vi "LDA_Analysis_1.vi"() -> (5 "Plug in titles":string[](array[string]), 7 "Plug in values":string[](array[string]))   [LabVIEW 2010]
uses:
  Globals/Plug_in_data_global.vi
  Globals/LDA_meas_global_1.vi
  Globals/Meas_global.vi
  Globals/Constants_global.vi
  Controls/Save_Data.ctl
  <vilib>/Analysis/NI_AALBase.lvlib
panel:
  in  "No of estimates output":i32=300
  out "Autocorrelation":cluster{dbl, dbl, dbl[]}[](graph)
  in  "Mode":T1(ring)
  in  "Separation Character":string="\t"
  in  "Precision":i16=2
  out "Ch names":string[](array[string])
  out "Number or Good blocks":i32
  out "Resampled block length":i32
  out "Resampling Frequency":dbl
  in  "Output Directory":path
  in  "File":T2=enum."Save Data"
  out "Frequency Spectrum":cluster{dbl, dbl, dbl[]}[](graph)
  # "You must have just these two indicators on the connector pane of the vi"
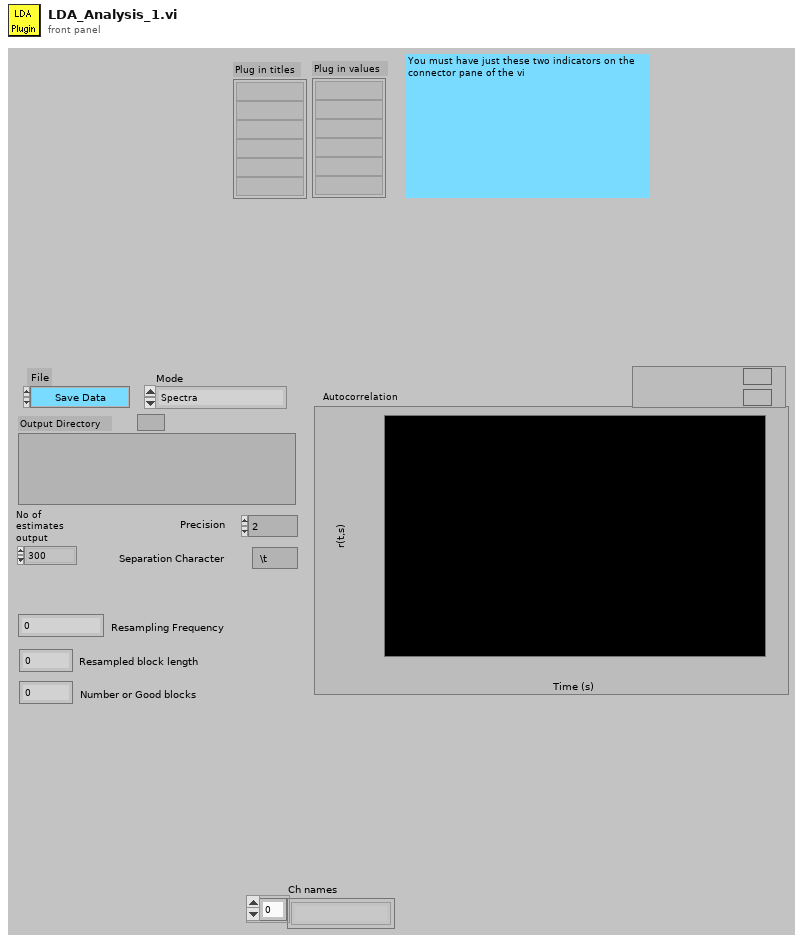
[diagram p1: front panel]
types:
  T1 = enum16{"Spectra", "Autocorrelation", "Calculate Error bars"}
  T2 = typedef "Save_Data.ctl" = enum16{"Save No Data", "Save Data"}
  T3 = enum32{"existing file", "new file", "new or existing file", "existing dir", "new dir", "new or existing dir", "existing file (use LLBs)", "new file (use LLBs)", "new or existing file (use LLBs)", "new or existing file or directory (use LLBs)"}
  T4 = typedef "Analysis_info_cluster.ctl" = cluster{"Colour":u32, "Inst type":T5, "Inst name":string, "Symbol":string, "Code name":string, "Extra Info":string, "Inst Array":T6, "Index":i32, "Voltage Index":i32, "Extra Titles":string[], "Extra Values":string[]}
  T5 = typedef "Inst_type.ctl" = enum16{"Propeller anemometer", "Raw voltage", "Pressure Transducer", "Pitot-static tube", "Preston tube", "Hot wire", "Cross wire 1", "Cross wire 2", "Generic Linear", "Generic Polynomial", "Generic BackPoly", "Fast FID", "Thermocouple", "Cold wire", "Pulsed Wire", "LDA Vel", "LDA Tran time", "LDA Arr time"}
  T6 = typedef "Instrument_Array.ctl" = enum16{"PWA", "LDA", "Analogue"}
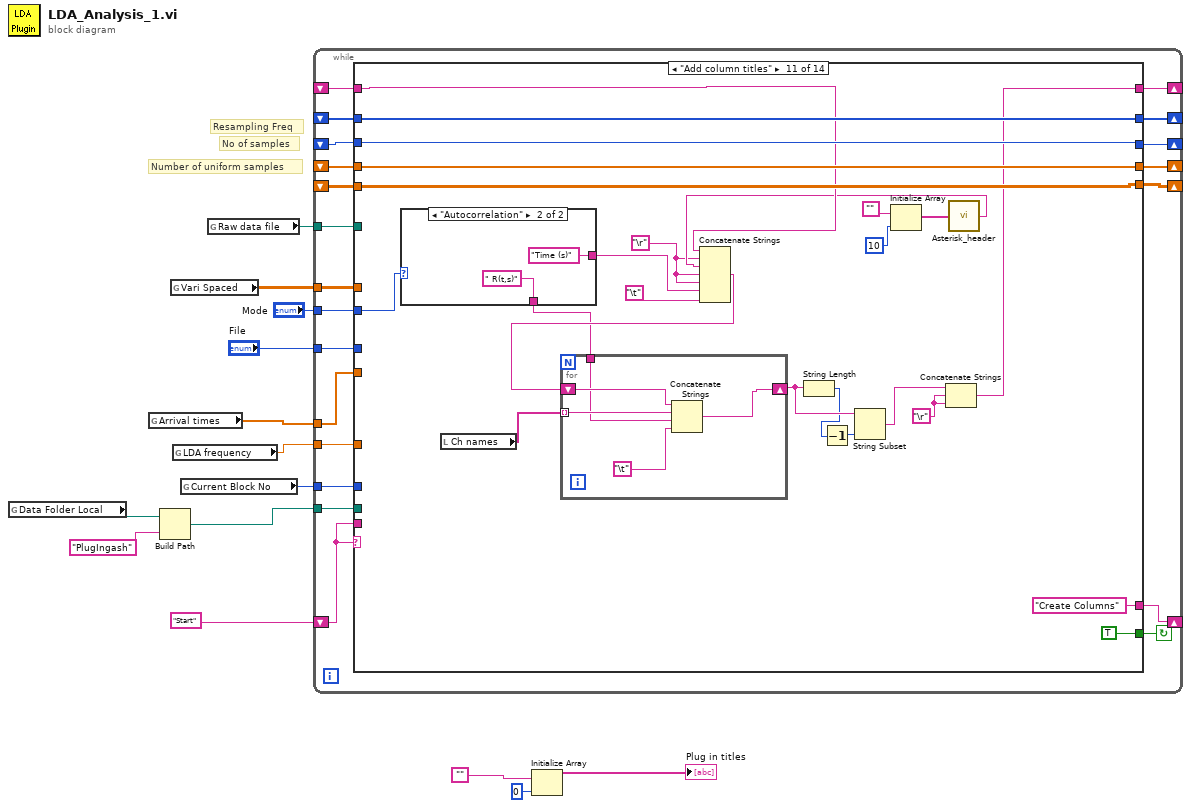
[diagram p0: block diagram]
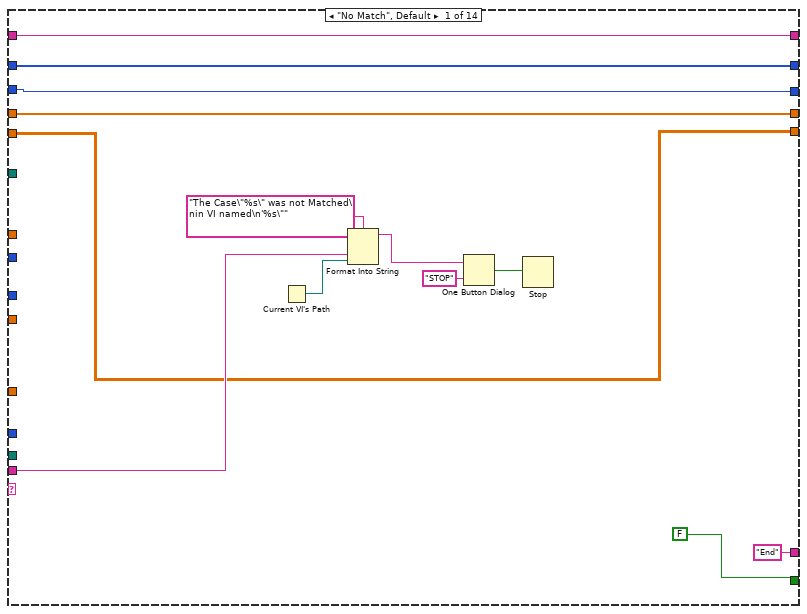
[diagram p2: hidden frame]
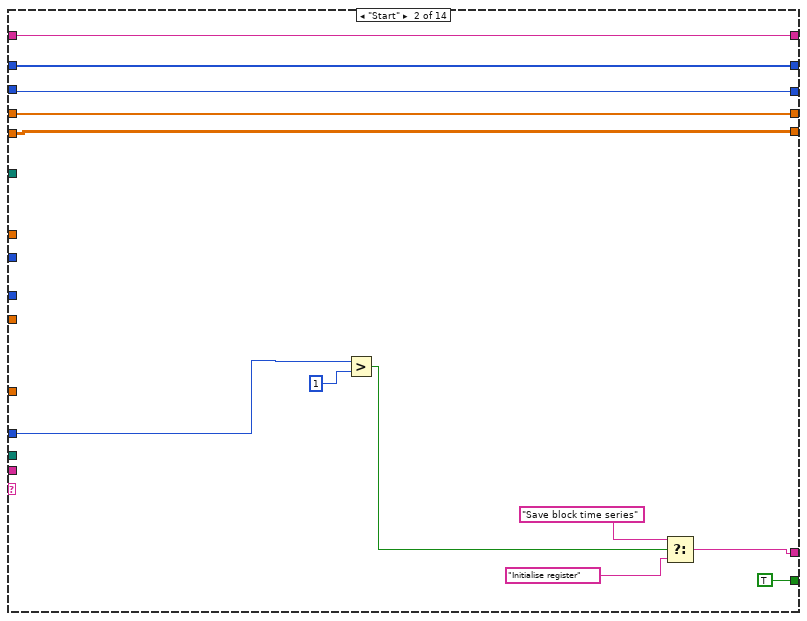
[diagram p3: hidden frame]
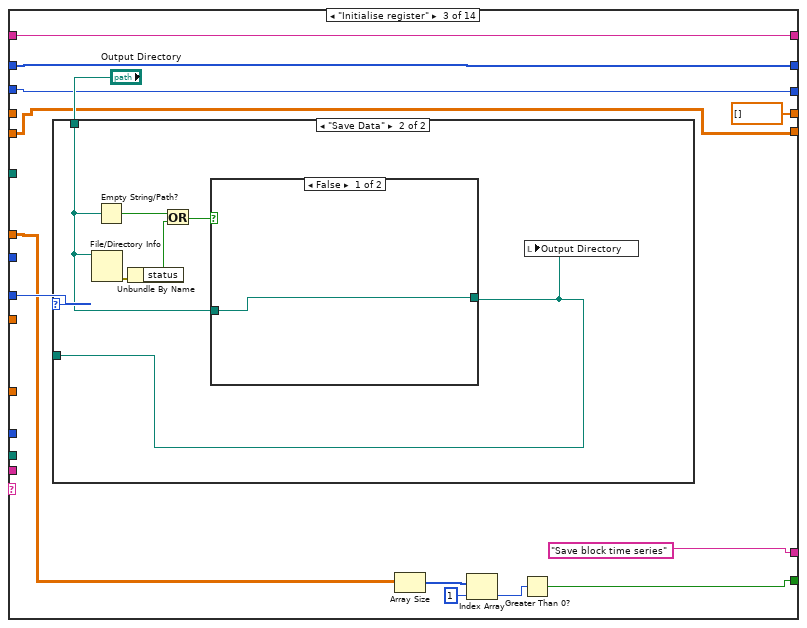
[diagram p4: hidden frame]
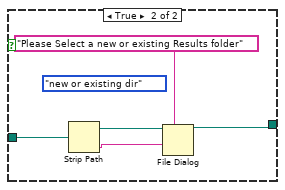
[diagram p6: hidden frame]
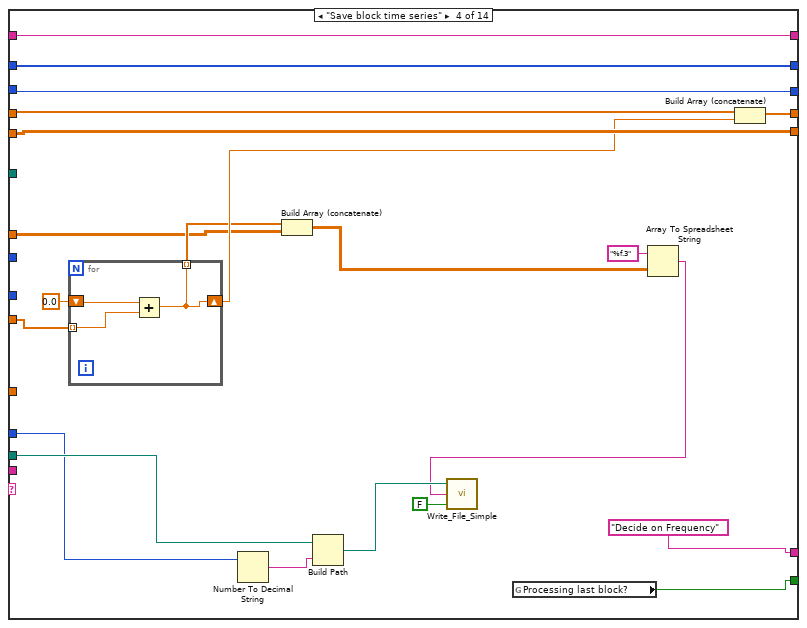
[diagram p7: hidden frame]
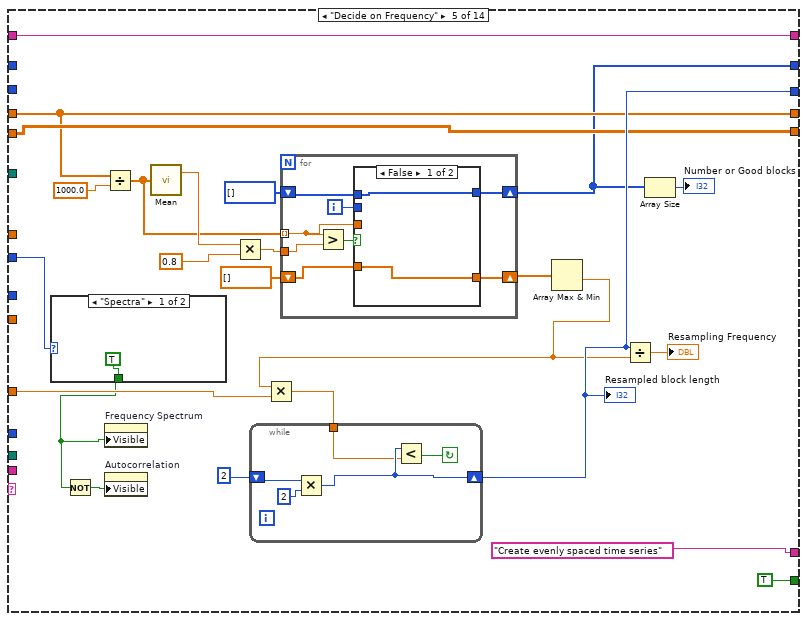
[diagram p8: hidden frame]
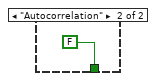
[diagram p9: hidden frame]
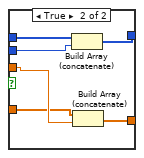
[diagram p10: hidden frame]
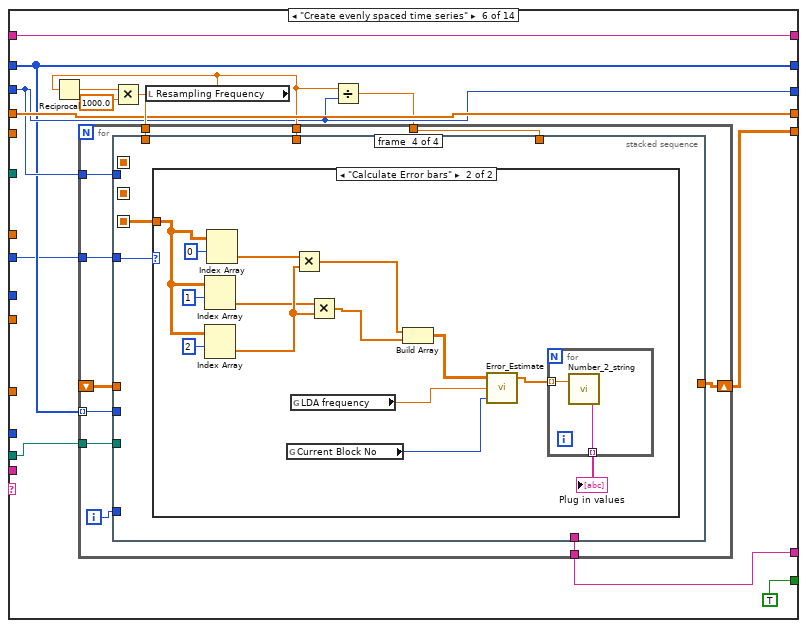
[diagram p11: hidden frame]
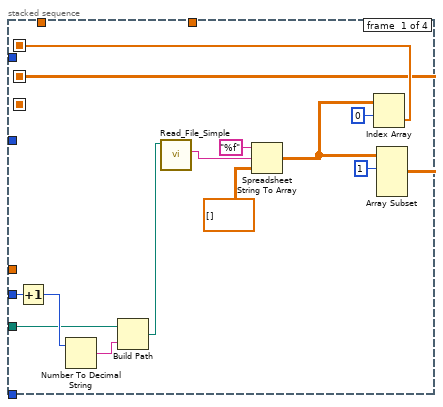
[diagram p12: hidden frame]
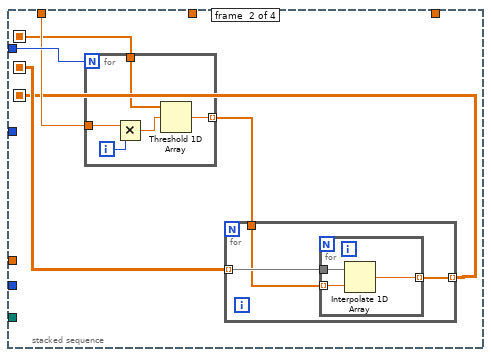
[diagram p13: hidden frame]
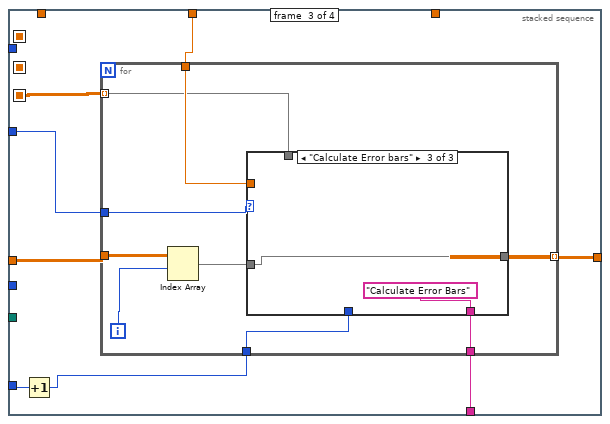
[diagram p14: hidden frame]
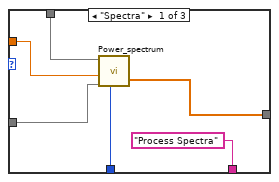
[diagram p15: hidden frame]
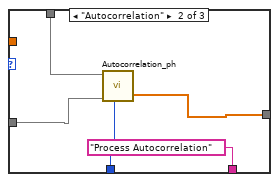
[diagram p16: hidden frame]
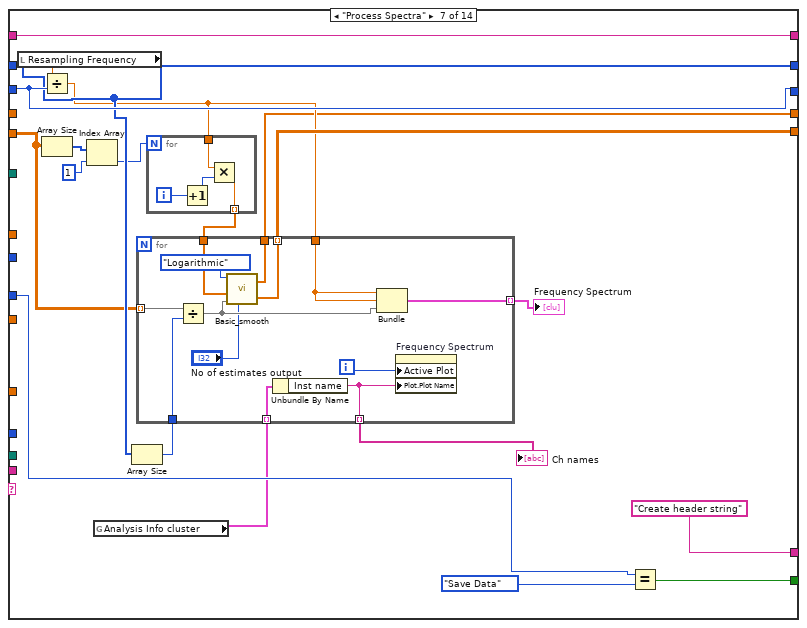
[diagram p18: hidden frame]
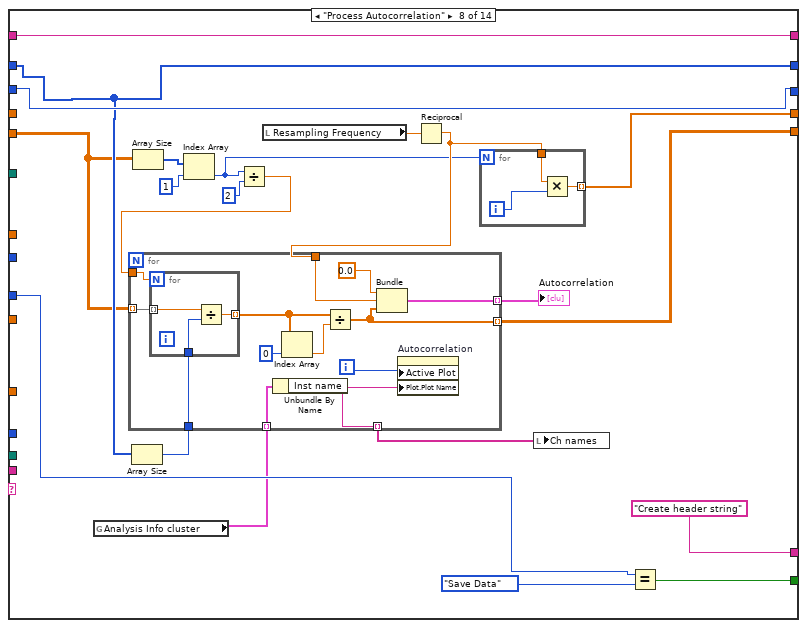
[diagram p19: hidden frame]
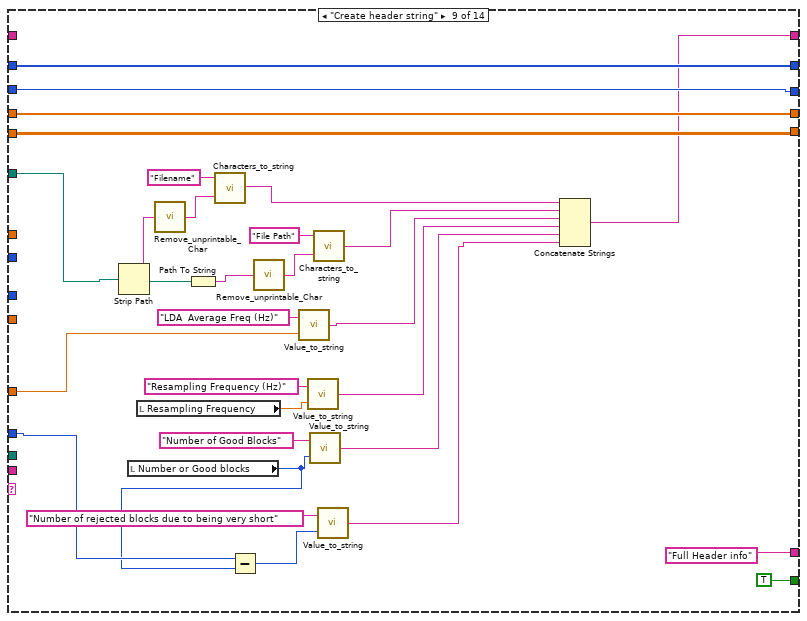
[diagram p20: hidden frame]
diagram:
  # "No of samples"
  # "Number of uniform samples"
  # "Resampling Freq"
  n1 = global read "Constants_global.vi" "Data Folder Local"() -> (w6:path)
  n2 = global read "LDA_meas_global_1.vi" "Arrival times"() -> (w12:dbl[])
  n3 = Build Path(base path=w6, name or relative path="PlugIngash") -> (appended path=w5:path)
  n4 = global read "Plug_in_data_global.vi" "Vari Spaced"() -> (w13:dbl[][])
  n5 = global read "Meas_global.vi" "LDA frequency"() -> (w2:dbl)
  n6 = global read "Meas_global.vi" "Current Block No"() -> (w8:i32)
  n7 = global read "Meas_global.vi" "Raw data file"() -> (w3:path)
  n8 = while {
    shift-left: "Start" -> [w35]
    shift-right: [w32] -> _
    tunnel: w13 -> [w34]
    tunnel: w12 -> [w33]
    shift-right: [w30] -> _
    shift-left: _ -> [w29]
    shift-right: [w28] -> _
    shift-left: _ -> [w27]
    tunnel: w8 -> [w26]
    tunnel: w5 -> [w25]
    shift-right: [w24] -> _
    shift-left: _ -> [w23]
    tunnel: "File" -> [w22]
    shift-right: [w21] -> _
    shift-left: _ -> [w20]
    tunnel: w3 -> [w19]
    tunnel: w2 -> [w18]
    shift-right: [w17] -> _
    shift-left: _ -> [w16]
    tunnel: "Mode" -> [w15]
    stop <- w31 continue-if-true
    n9 = case shown="\"Add column titles\"" w35 {
      tunnel: ["End" ("t") w55 "Save block time series" ("t") "Decide on Frequency" ("t") "Create evenly spaced time series" ("t") w158 "Create header string" "Create header string" "Full Header info" ("t") "Add column titles" ("t") "Create Columns" ("t") "Save to file" ("t") "End" ("t") "End" ("t")] -> w32
      tunnel: w35 -> [w44 _ _ _ _ _ _ _ _ _ _ _ _ _]
      tunnel: w34 -> [_ _ w65 w89 _ _ _ _ _ _ _ _ _ _]
      tunnel: w33 -> [_ _ _ w93 _ _ _ _ _ _ _ _ _ _]
      tunnel: [FALSE TRUE w61 w99 TRUE TRUE ("Processing last block?") w274 w314 TRUE ("Processing last block?") TRUE ("Processing last block?") TRUE ("Processing last block?") TRUE ("Processing last block?") FALSE FALSE] -> w31
      tunnel: [w41 w51 w68 w94 w127 w167 w270 w308 w341 w376 w400 w418 _ _] -> w30
      tunnel: w29 -> [w41 w51 w68 w94 w127 _ w262 w305 w341 w376 w400 w418 _ _]
      tunnel: [w39 w54 dbl[] [] w97 w123 w166 w265 w299 w342 w377 w401 w413 w472 w500] -> w28
      tunnel: w27 -> [w39 w54 _ w98 w123 w166 _ _ w342 w377 w401 w413 w472 w500]
      tunnel: w26 -> [_ w53 _ w104 _ _ _ _ w350 _ _ _ _ _]
      tunnel: w25 -> [_ _ _ w105 _ w169 _ _ _ _ _ _ _ _]
      tunnel: [w40 w52 w69 w95 w128 w163 w277 w317 w343 w378 w402 w420 w473 w501] -> w24
      tunnel: w23 -> [w40 w52 w69 w95 _ w163 w277 w317 w343 w378 w402 w420 w473 w501]
      tunnel: w22 -> [_ _ w70 _ _ _ w275 w315 _ _ _ _ _ _]
      tunnel: [w38 w50 w67 w88 w117 w161 w269 w311 w344 w379 w403 w428 w471 w499] -> w21
      tunnel: w20 -> [w38 w50 w67 w88 _ w161 w269 w311 w344 w379 w403 w428 w471 w499]
      tunnel: w19 -> [_ _ _ _ _ _ _ _ w356 w369 _ _ w470 _]
      tunnel: w18 -> [_ _ _ _ w115 _ _ _ w353 _ _ _ _ _]
      tunnel: [w37 w49 w66 w87 w114 w160 w273 w313 w340 w368 w396 w424 w462 w498] -> w17
      tunnel: w16 -> [w37 w49 w66 w87 w114 w160 w273 w313 _ w375 w390 w425 w462 w498]
      tunnel: w15 -> [_ _ _ _ w113 w159 _ _ _ _ w393 _ w459 _]
      frame "No Match", Default {
        n10 = Current VI's Path() -> (path=w43:path)
        n11 = Format Into String(format string="The Case\"%s\" was not Matched\nin VI named\n'%s\"" ("Format String"), w44, w43) -> (resulting string=w47:string)  [unwired: 2 in, 1 out]
        n12 = One Button Dialog(message=w47, button name ("OK")="STOP") -> (true=w45:bool)
        n13 = Stop(stop? (T)=w45) -> ()
      }
      frame "Start" {
        n14 = Greater?(x=w53, y=1) -> (0:w57:bool)
        n15 = Select(t="Save block time series", s=w57, f="Initialise register") -> (s? t:f=w55:string)
      }
      frame "Initialise register" {
        n16 = case shown="\"Save Data\"" w70 {
          tunnel: [w74 w80] -> _
          tunnel: "Output Directory" -> [w74 w78]
          frame "Save No Data" {
          }
          frame "Save Data" {
            n17 = File/Directory Info(path=w78) -> (error out=w79:errorcluster)  [unwired: 1 in, 6 out]
            n18 = Empty String/Path?(string/path=w78) -> (empty?=w76:bool)
            n19 = Unbundle By Name(w79) -> ("status"=w77:bool)
            n20 = Or(x=w76, y=w77) -> (x .or. y?=w75:bool)
            n21 = case shown="False" w75 {
              tunnel: [w81 w86] -> w80
              tunnel: w78 -> [w81 w84]
              frame False {
              }
              frame True {
                (unwired) T3."new or existing dir" ("select mode (2)")
                n22 = Strip Path(path=w84) -> (stripped path=w83:path, name=w82:string)
                n23 = File Dialog(7:"Please Select a new or existing Results folder" ("prompt"), 9:w82, 11:w83) -> (3:w86:path)  [unwired: 1 in, 6 out]
              }
            }
            n24 = local write "Output Directory"(w80) -> ()
          }
        }
        n25 = Array Size(array=w65) -> (size(s)=w64:i32[])
        n26 = Index Array(array=w64, index=1) -> (element=w62:i32)
        n27 = Greater Than 0?(x=w62) -> (x > 0?=w61:bool)
      }
      frame "Save block time series" {
        n28 = for {
          shift-right: [w108] -> w91
          shift-left: 0.0 -> [w110]
          tunnel: w93 -> [w109] mode=indexing
          tunnel: [w108] -> w90 mode=indexing
          n29 = Add(x=w110, y=w109) -> (x+y=w108:dbl)
        }
        n30 = Number To Decimal String(number=w104) -> (decimal integer string=w103:string)  [unwired: 1 out]
        n31 = Build Array (concatenate)(w90, w89) -> (w96:dbl[][])
        n32 = Build Path(base path=w105, name or relative path=w103) -> (appended path=w102:path)
        n33 = global read "Meas_global.vi" "Processing last block?"() -> (w99:bool)
        n34 = Array To Spreadsheet String(array=w96, 3:"%f.3" ("format string")) -> (spreadsheet string=w101:string)  [unwired: 1 out]
        n35 = call "Write_File_Simple.vi"("append to file? (new file:F)"=FALSE, "character string"=w101, "file path"=w102) -> ()  [unwired: 2 out]
        n36 = Build Array (concatenate)(w98, w91) -> (w97:dbl[])
      }
      frame "Decide on Frequency" {
        n37 = case shown="\"Spectra\"" w113 {
          tunnel: [TRUE FALSE] -> w111
          frame "Spectra" {
          }
          frame "Autocorrelation" {
          }
        }
        n38 = Not(x=w111) -> (.not. x?=w112:bool)
        n39 = Divide(x=w123, y=1000.0) -> (x/y=w121:dbl[])
        n40 = property on="Frequency Spectrum" class="WFGraph (strict)"("Visible"=w111) -> ()  [unwired: 2 in, 2 out]
        n41 = property on="Autocorrelation" class="WFGraph (strict)"("Visible"=w112) -> ()  [unwired: 2 in, 2 out]
        n42 = call <vilib>:"Mean.vi"("X"=w121) -> ("mean"=w126:dbl)  [unwired: 1 out]
        n43 = Multiply(x=w126, y=0.8) -> (x*y=w124:dbl)
        n44 = for {
          tunnel: w121 -> [w139] mode=indexing
          tunnel: w124 -> [w144]
          shift-right: [w140] -> w117
          shift-left: i32[] [] -> [w141]
          shift-right: [w137] -> w119
          shift-left: dbl[] [] -> [w138]
          i -> [w142]
          n45 = Greater?(x=w139, y=w144) -> (0:w143:bool)
          n46 = case shown="False" w143 {
            tunnel: w142 -> [_ w152]
            tunnel: w141 -> [w146 w151]
            tunnel: [w146 w150] -> w140
            tunnel: w139 -> [_ w149]
            tunnel: w138 -> [w145 w148]
            tunnel: [w145 w147] -> w137
            frame False {
            }
            frame True {
              n47 = Build Array (concatenate)(w151, w152) -> (w150:i32[])
              n48 = Build Array (concatenate)(w148, w149) -> (w147:dbl[])
            }
          }
        }
        n49 = Array Max & Min(array=w119) -> (min value=w118:dbl)  [unwired: 3 out]
        n50 = Multiply(x=w118, y=w115) -> (x*y=w130:dbl)
        n51 = while {
          shift-right: [w155] -> w128
          shift-left: 2 -> [w157]
          tunnel: w130 -> [w154]
          stop <- w153 continue-if-true
          n52 = Multiply(x=w157, y=2) -> (x*y=w155:i32)
          n53 = Less?(x=w155, y=w154) -> (x < y?=w153:bool)
        }
        "Resampled block length" <- w128
        n54 = Divide(x=w128, y=w118) -> (x/y=→"Resampling Frequency":dbl)
        n55 = Array Size(array=w117) -> (size(s)=→"Number or Good blocks":i32)
      }
      frame "Create evenly spaced time series" {
        n56 = local read "Resampling Frequency"() -> (w164:dbl)
        n57 = Reciprocal(x=w164) -> (1/x=w170:dbl)
        n58 = Multiply(x=w170, y=1000.0) -> (x*y=w168:dbl)
        n59 = Divide(x=w164, y=w163) -> (x/y=w162:dbl)
        n60 = for {
          tunnel: w169 -> [w182]
          tunnel: w163 -> [w181]
          tunnel: w168 -> [w180]
          shift-right: [w178] -> w167
          shift-left: _ -> [w179]
          tunnel: w164 -> [w177]
          tunnel: w162 -> [w176]
          tunnel: w161 -> [w174] mode=indexing
          tunnel: w159 -> [w173]
          tunnel: [w172] -> w158
          i -> [w175]
          n61 = stacked-sequence {
            seq-local: [w188 _ _ _] -> [_ w199 _ _]
            seq-local: [w185 _ _ _] -> [_ w197 _ _]
            seq-local: [_ w196 _ _] -> [_ _ w220 w244]
            tunnel: w175 -> [_ _ w216 _]
            tunnel: w182 -> [w193 _ _ _]
            tunnel: w181 -> [_ w201 _ _]
            tunnel: w180 -> [_ w200 _ _]
            tunnel: w179 -> [_ _ w219 _]
            tunnel: [_ _ w218 _] -> w178
            tunnel: w177 -> [_ _ w217 _]
            tunnel: w176 -> [_ _ _ _]
            tunnel: w174 -> [w183 _ _ _]
            tunnel: w173 -> [_ _ w214 w243]
            tunnel: [_ _ w213 _] -> w172
            frame #0 {
              n62 = Increment(x=w183) -> (x+1=w194:i32)
              n63 = Number To Decimal String(number=w194) -> (decimal integer string=w195:string)  [unwired: 1 out]
              n64 = Build Path(base path=w193, name or relative path=w195) -> (appended path=w192:path)
              n65 = call "Read_File_Simple.vi"("Filename"=w192) -> ("string"=w191:string)  [unwired: 2 in, 7 out]
              n66 = Spreadsheet String To Array(format string="%f", spreadsheet string=w191, array type (2D Dbl)=dbl[][] []) -> (array=w187:dbl[][])  [unwired: 1 out]
              n67 = Index Array(array=w187, index (row)=0) -> (element=w188:dbl[])  [unwired: 1 in]
              n68 = Array Subset(array=w187, index (row)=1 ("index")) -> (w185:dbl[][])  [unwired: 3 in]
            }
            frame #1 {
              n69 = for {
                N: w201 -> [_]
                tunnel: w200 -> [w211]
                tunnel: w199 -> [w209]
                tunnel: [w208] -> w198 mode=indexing
                i -> [w212]
                n70 = Multiply(x=w211, y=w212) -> (x*y=w210:dbl)
                n71 = Threshold 1D Array(2:w210, 3:w209) -> (0:w208:dbl)  [unwired: 1 out]
              }
              n72 = for {
                tunnel: [w204] -> w196 mode=indexing
                tunnel: w198 -> [w202]
                tunnel: w197 -> [w203] mode=indexing
                n73 = for {
                  tunnel: w203 -> [w207]
                  tunnel: w202 -> [w206] mode=indexing
                  tunnel: [w205] -> w204 mode=indexing
                  n74 = Interpolate 1D Array(1:w206, 2:w207) -> (0:w205:dbl)
                }
              }
            }
            frame #2 {
              n75 = Increment(x=w216) -> (x+1=w215:i32)
              n76 = for {
                tunnel: w220 -> [w225] mode=indexing
                tunnel: [w224] -> w218 mode=indexing
                tunnel: w219 -> [w229]
                tunnel: w217 -> [w226]
                tunnel: w215 -> [w223]
                tunnel: w214 -> [w222]
                tunnel: [w221] -> w213
                i -> [w227]
                n77 = Index Array(array=w229, index (row)=w227) -> (element=w228:dbl[])  [unwired: 1 in]
                n78 = case shown="\"Calculate Error bars\"" w222 {
                  tunnel: w228 -> [w235 w239 w242]
                  tunnel: w226 -> [w234 _ _]
                  tunnel: w225 -> [w233 w240 _]
                  tunnel: [w232 w238 w242] -> w224
                  tunnel: w223 -> [w231 w237 _]
                  tunnel: ["Process Spectra" ("t") "Process Autocorrelation" ("t") "Calculate Error Bars" ("t")] -> w221
                  frame "Spectra" {
                    n79 = call "Power_spectrum.vi"("U"=w233, "Sampling frequency"=w234, "Spectrum input array"=w235, "Block No"=w231) -> ("Spectrum output array"=w232:dbl[])  [unwired: 1 in, 1 out]
                  }
                  frame "Autocorrelation" {
                    n80 = call "Autocorrelation_ph.vi"("X"=w240, "Autocorrelation of X"=w239, "Block No"=w237) -> ("Autocorrelation of X"=w238:dbl[])  [unwired: 2 in, 1 out]
                  }
                  frame "Calculate Error bars" {
                  }
                }
              }
            }
            frame #3 {
              n81 = case shown="\"Calculate Error bars\"" w243 {
                tunnel: w244 -> [_ w247]
                frame "Spectra", Default {
                }
                frame "Calculate Error bars" {
                  n82 = Index Array(array=w247, index (row)=1) -> (element=w252:dbl[])  [unwired: 1 in]
                  n83 = Index Array(array=w247, index (row)=2) -> (element=w253:dbl[])  [unwired: 1 in]
                  n84 = Index Array(array=w247, index (row)=0) -> (element=w251:dbl[])  [unwired: 1 in]
                  n85 = global read "Meas_global.vi" "Current Block No"() -> (w249:i32)
                  n86 = global read "Meas_global.vi" "LDA frequency"() -> (w248:dbl)
                  n87 = Multiply(x=w251, y=w253) -> (x*y=w254:dbl[])
                  n88 = Multiply(x=w252, y=w253) -> (x*y=w255:dbl[])
                  n89 = Build Array(w254, w255) -> (w250:dbl[][])
                  n90 = call "Error_Estimate.vi"("Block No"=w249, "Sampling Frequency (Hz)"=w248, "Data In"=w250) -> ("Error Estimates"=w246:dbl[])  [unwired: 2 out]
                  n91 = for {
                    tunnel: w246 -> [w260] mode=indexing
                    tunnel: [w259] -> w245 mode=indexing
                    n92 = call "Number_2_string.vi"("number"=w260) -> ("String"=w259:string)  [unwired: 1 in]
                  }
                  "Plug in values" <- w245
                }
              }
            }
          }
        }
      }
      frame "Process Spectra" {
        (unwired) FALSE
        n93 = local read "Resampling Frequency"() -> (w278:dbl)
        n94 = Divide(x=w278, y=w277) -> (x/y=w267:dbl)
        n95 = Array Size(array=w262) -> (size(s)=w264:i32[])
        n96 = Index Array(array=w264, index=1) -> (element=w261:i32)
        n97 = global read "Meas_global.vi" "Analysis Info cluster"() -> (w271:T4[])
        n98 = Array Size(array=w269) -> (size(s)=w268:i32)
        n99 = for {
          N: w261 -> [_]
          tunnel: w267 -> [w282]
          tunnel: [w281] -> w266 mode=indexing
          i -> [w284]
          n100 = Increment(x=w284) -> (x+1=w283:i32)
          n101 = Multiply(x=w282, y=w283) -> (x*y=w281:dbl)
        }
        n102 = for {
          tunnel: w267 -> [w297]
          tunnel: w262 -> [w296] mode=indexing
          tunnel: w268 -> [w295]
          tunnel: [w294] -> w279 mode=indexing
          tunnel: w271 -> [w292] mode=indexing
          tunnel: [w291] -> w272 mode=indexing
          tunnel: [w286] -> w270 mode=indexing
          tunnel: w266 -> [w289]
          tunnel: [w285] -> w265
          i -> [w293]
          n103 = Divide(x=w296, y=w295) -> (x/y=w290:dbl[])
          n104 = call "Basic_smooth.vi"("Smoothing"=enum16{"Linear", "Logarithmic"}."Logarithmic", "X array in"=w289, "Y array in"=w290, "No of estimates output"="No of estimates output") -> ("X array Out"=w285:dbl[], "Y array Out"=w286:dbl[])  [unwired: 1 out]
          n105 = Unbundle By Name(w292) -> ("Inst name"=w291:string)
          n106 = Bundle(w297, w297, w290) -> (w294:cluster{dbl, dbl, dbl[]})  [unwired: 1 out]
          n107 = property on="Frequency Spectrum" class="WFGraph (strict)"("Active Plot"=w293, "Plot.Plot Name"=w291) -> ()  [unwired: 2 in, 2 out]
        }
        "Frequency Spectrum" <- w279
        "Ch names" <- w272
        n108 = Equal?(x=w275, y=Save_Data."Save Data" ("File")) -> (x = y?=w274:bool)
      }
      frame "Process Autocorrelation" {
        (unwired) FALSE
        n109 = global read "Meas_global.vi" "Analysis Info cluster"() -> (w312:T4[])
        n110 = Array Size(array=w311) -> (size(s)=w310:i32)
        n111 = Array Size(array=w305) -> (size(s)=w304:i32[])
        n112 = Index Array(array=w304, index=1) -> (element=w298:i32)
        n113 = Divide(x=w298, y=2) -> (x/y=w301:dbl)
        n114 = local read "Resampling Frequency"() -> (w309:dbl)
        n115 = Reciprocal(x=w309) -> (1/x=w300:dbl)
        n116 = for {
          tunnel: w300 -> [w334]
          tunnel: w305 -> [w333] mode=indexing
          tunnel: w310 -> [w332]
          tunnel: [w331] -> w306 mode=indexing
          tunnel: w312 -> [w330] mode=indexing
          tunnel: [w325] -> w308 mode=indexing
          tunnel: [w323] -> w307 mode=indexing
          tunnel: w301 -> [w322]
          i -> [w324]
          n117 = for {
            N: w322 -> [_]
            tunnel: w333 -> [w337] mode=indexing
            tunnel: w332 -> [w336]
            tunnel: [w335] -> w327 mode=indexing
            n118 = Divide(x=w337, y=w336) -> (x/y=w335:dbl)
          }
          n119 = Unbundle By Name(w330) -> ("Inst name"=w323:string)
          n120 = Index Array(array=w327, index=0) -> (element=w326:dbl)
          n121 = Divide(x=w327, y=w326) -> (x/y=w325:dbl[])
          n122 = Bundle(0.0, w334, w325) -> (w331:cluster{dbl, dbl, dbl[]})  [unwired: 1 out]
          n123 = property on="Autocorrelation" class="WFGraph (strict)"("Active Plot"=w324, "Plot.Plot Name"=w323) -> ()  [unwired: 2 in, 2 out]
        }
        "Autocorrelation" <- w306
        n124 = for {
          N: w298 -> [_]
          tunnel: w300 -> [w321]
          tunnel: [w319] -> w299 mode=indexing
          i -> [w320]
          n125 = Multiply(x=w321, y=w320) -> (x*y=w319:dbl)
        }
        n126 = local write "Ch names"(w307) -> ()
        n127 = Equal?(x=w315, y=Save_Data."Save Data" ("File")) -> (x = y?=w314:bool)
      }
      frame "Create header string" {
        n128 = Strip Path(path=w356) -> (stripped path=w360:path, name=w364:string)
        n129 = local read "Number or Good blocks"() -> (w349:i32)
        n130 = local read "Resampling Frequency"() -> (w352:dbl)
        n131 = call "Remove_unprintable_Char.vi"("Input String"=w364) -> ("Output String"=w363:string)
        n132 = Path To String(path=w360) -> (string=w359:string)
        n133 = call "Characters_to_string.vi"("Characters to write"=w363, "Label for characters"="Filename") -> ("Output string"=w358:string)
        n134 = Subtract(x=w350, y=w349) -> (x-y=w348:i32)
        n135 = call "Remove_unprintable_Char.vi"("Input String"=w359) -> ("Output String"=w362:string)
        n136 = call "Value_to_string.vi"("Value"=w353, "Label for value"="LDA  Average Freq (Hz)") -> ("Output string"=w367:string)  [unwired: 1 in]
        n137 = call "Value_to_string.vi"("Value"=w352, "Label for value"="Resampling Frequency (Hz)") -> ("Output string"=w347:string)  [unwired: 1 in]
        n138 = call "Value_to_string.vi"("Value"=w349, "Label for value"="Number of Good Blocks") -> ("Output string"=w346:string)  [unwired: 1 in]
        n139 = call "Characters_to_string.vi"("Characters to write"=w362, "Label for characters"="File Path") -> ("Output string"=w357:string)
        n140 = call "Value_to_string.vi"("Value"=w348, "Label for value"="Number of rejected blocks due to being very short") -> ("Output string"=w345:string)  [unwired: 1 in]
        n141 = Concatenate Strings(w358, w357, w367, w347, w346, w345) -> (w340:string)
      }
      frame "Full Header info" {
        w372 = "\r"
        n142 = call "Read_RD_Ch_header.vi"("Raw data file"=w369) -> ("Ch string"=w370:string)  [unwired: 3 out]
        n143 = Concatenate Strings(w375, w372, "*****This is a many rows per single point file*****", w372, w370) -> (w368:string)
      }
      frame "Add column titles" {
        w384 = "\r"
        w385 = "\r"
        n144 = case shown="\"Autocorrelation\"" w393 {
          tunnel: ["f (Hz)" "Time (s)"] -> w392
          tunnel: [" E(f)" " R(t,s)"] -> w391
          frame "Spectra" {
          }
          frame "Autocorrelation" {
          }
        }
        n145 = local read "Ch names"() -> (w398:string[])
        n146 = Initialize Array("", 10) -> (w389:string[])
        n147 = call "Asterisk_header.vi"("Channel names"=w389) -> ("Header string"=w386:string)
        n148 = Concatenate Strings(w390, w384, w386, w384, w384, w392, "\t") -> (w397:string)
        n149 = for {
          shift-right: [w409] -> w383
          shift-left: w397 -> [w411]
          tunnel: w398 -> [w412] mode=indexing
          tunnel: w391 -> [w408]
          n150 = Concatenate Strings(w411, w412, w408, "\t") -> (w409:string)
        }
        n151 = String Length(string=w383) -> (length=w380:i32)
        n152 = Decrement(x=w380) -> (x-1=w381:i32)
        n153 = String Subset(string=w383, length (rest)=w381) -> (substring=w382:string)  [unwired: 1 out]
        n154 = Concatenate Strings(w382, w385, w385) -> (w396:string)
      }
      frame "Create Columns" {
        n155 = Array Size(array=w418) -> (size(s)=w416:i32[])
        n156 = Index Array(array=w416, index=0) -> (element=w415:i32)
        n157 = Decrement(x=w415) -> (x-1=w414:i32)
        n158 = for {
          shift-right: [w442] -> w423
          shift-left: "" -> [w437]
          tunnel: "Separation Character" -> [w430]
          tunnel: w418 -> [w440]
          tunnel: w414 -> [w436]
          tunnel: "Precision" -> [w434]
          tunnel: "Precision" -> [w433]
          tunnel: w413 -> [w429] mode=indexing
          i -> [w435]
          n159 = Index Array(array=w440, index (col)=w435) -> (element=w439:dbl[])  [unwired: 1 in]
          n160 = Number To Fractional String(number=w429, precision (6)=w433) -> (F-format string=w432:string)  [unwired: 2 out]
          n161 = Concatenate Strings(w432, w430) -> (w431:string)
          n162 = for {
            shift-right: [w449] -> w438
            shift-left: w431 -> [w451]
            tunnel: w430 -> [w448]
            tunnel: w439 -> [w443] mode=indexing
            tunnel: w436 -> [w446]
            tunnel: w434 -> [w444]
            i -> [w447]
            n163 = Equal?(x=w447, y=w446) -> (x = y?=w445:bool)
            n164 = Number To Exponential String(number=w443, precision (6)=w444) -> (E-format string=w450:string)  [unwired: 2 out]
            n165 = case shown="True" w445 {
              tunnel: w451 -> [w455 w458]
              tunnel: w450 -> [w454 w457]
              tunnel: [w453 w456] -> w449
              tunnel: w448 -> [w452 _]
              frame False {
                n166 = Concatenate Strings(w455, w454, w452) -> (w453:string)
              }
              frame True {
                n167 = Concatenate Strings(w458, w457) -> (w456:string)
              }
            }
          }
          n168 = Concatenate Strings(w437, w438, "\r") -> (w442:string)
        }
        n169 = Concatenate Strings(w425, w423) -> (w424:string)
      }
      frame "Save to file" {
        w464 = TRUE  # advisory dialog? (display:T)
        n170 = case shown="\"Autocorrelation\"" w459 {
          tunnel: ["Spec_" ("string") "Auto_" ("string")] -> w460
          frame "Spectra" {
          }
          frame "Autocorrelation" {
          }
        }
        n171 = Strip Path(path=w470) -> (name=w468:string)  [unwired: 1 out]
        n172 = local read "Output Directory"() -> (w469:path)
        n173 = Concatenate Strings(w460, w468) -> (w467:string)
        n174 = Build Path(base path=w469, name or relative path=w467) -> (appended path=w466:path)
        n175 = call "Create_directory_path.vi"("Path name"=w466) -> ("Path name Out"=w465:path)
        n176 = call "Write_Characters_To_File.vi"("file path (dialog if empty)"=w465, "advisory dialog? (display:T)"=w464, "character string"=w462, "append to file? (new file:F)"=FALSE) -> ()  [unwired: 1 in, 4 out]
      }
      frame "Calculate Error Bars" {
        w486 = 2 ("index (row)")
        w487 = 1 ("index (row)")
        w485 = 0 ("index (row)")
        n177 = global read "Meas_global.vi" "Analysis Info cluster"() -> (w494:T4[])
        n178 = Index Array(index (row)=w487) -> (array=w479:dbl[][], element=w481)  [unwired: 1 in]
        n179 = Index Array(index (row)=w486) -> (array=w478:dbl[][], element=w482)  [unwired: 1 in]
        n180 = Index Array(index (row)=w485) -> (element=w480)  [unwired: 2 in]
        n181 = Index Array(index=w485) -> (array=w488:string[], element=w489)
        n182 = Index Array(array=w488, index=w486) -> (element=w491)
        n183 = for {
          tunnel: w494 -> [w507] mode=indexing
          tunnel: [w506] -> w495 mode=indexing
          tunnel: [w505] -> _ mode=indexing
          tunnel: [w504] -> _ mode=indexing
          tunnel: [w503] -> w496 mode=indexing
          n184 = Unbundle By Name(w507) -> ("Symbol"=w503:string, "Inst name"=w506:string, "Index"=w504:i32, "Inst Array"=w505:T6)
        }
        n185 = Multiply(x=w480, y=w482) -> (x*y=w483:dbl)
        n186 = Multiply(x=w481, y=w482) -> (x*y=w484:dbl)
        n187 = Index Array(array=w488, index=w487) -> (element=w492)
        n188 = Concatenate Strings(w489, w491) -> (w490:string)
        n189 = Concatenate Strings(w492, w491) -> (w493:string)
        n190 = Build Array(w483, w484) -> (w477:dbl[])
      }
    }
  }
  n191 = Initialize Array("", 0) -> (→"Plug in titles":string[])
